vi "equals array.vi"(8 "y":dbl[](array[numeric]), 10 "x":dbl) -> (2 "x = y?":bool)   [LabVIEW 2010]
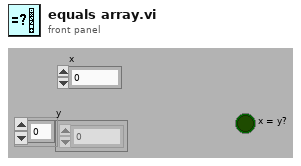
[diagram p1: front panel]
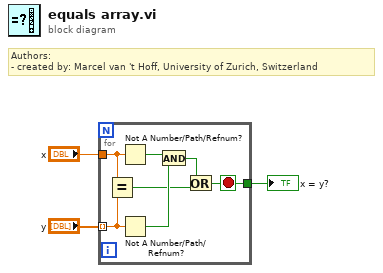
[diagram p0: block diagram]
diagram:
  # "Authors: \n- created by: Marcel van 't Hoff, University of Zurich, Switzerland"
  n1 = for {
    tunnel: "y" -> [w10] mode=indexing
    tunnel: "x" -> [w9]
    tunnel: [w4] -> w3
    stop <- w4 stop-if-true
    n2 = Equal?(x=w9, y=w10) -> (x = y?=w5:bool)
    n3 = Not A Number/Path/Refnum?(number/path/refnum=w9) -> (NaN/Path/Refnum?=w8:bool)
    n4 = Not A Number/Path/Refnum?(number/path/refnum=w10) -> (NaN/Path/Refnum?=w7:bool)
    n5 = And(x=w8, y=w7) -> (x .and. y?=w6:bool)
    n6 = Or(x=w6, y=w5) -> (x .or. y?=w4:bool)
  }
  "x = y?" <- w3
